vi "Part 2.vi"(11 "Input":string) -> (3 "Output":i64)   [LabVIEW 2021]
uses:
  <userlib>/_OpenG.lib/string/string.llb/Convert EOLs (String)__ogtk.vi
  0a5bc26e-a1a3-4762-95bb-f84fbea421ee.vi
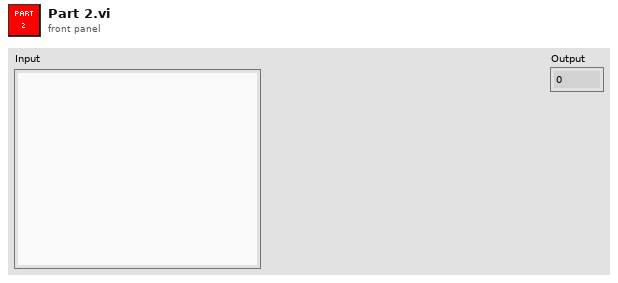
[diagram p1: front panel]
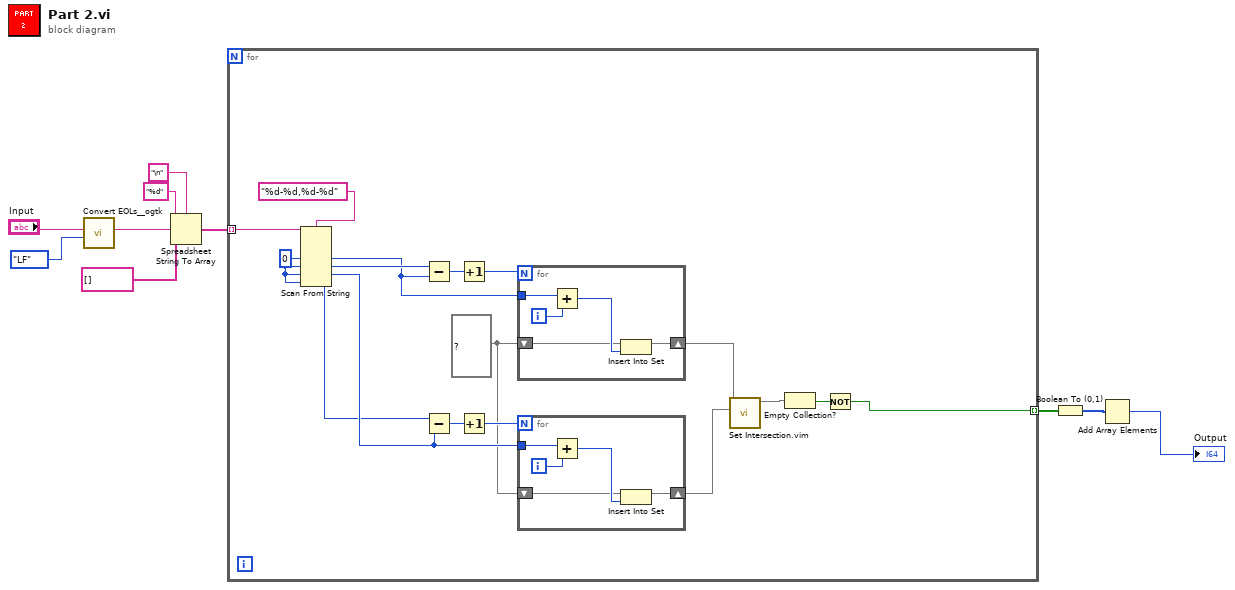
[diagram p0: block diagram]
diagram:
  n1 = call-poly <userlib>:"Convert EOLs__ogtk.vi"("Convert to:"=enum16{"CR", "LF", "CRLF"}."LF", "String in"="Input") -> ("String out"=w7:string)  [unwired: 9 in]
  n2 = Spreadsheet String To Array(delimiter (Tab)="\n", format string="%d", spreadsheet string=w7, array type (2D Dbl)=string[] []) -> (array=w5:string[])
  n3 = for {
    tunnel: w5 -> [w27] mode=indexing
    tunnel: [w11] -> w4 mode=indexing
    w16 = set{i64} {} ("set out")
    w25 = i64 0 ("default value 1")
    n4 = Scan From String(format string="%d-%d,%d-%d", input string=w27, default 1=w25, default 2=w25, default 3=w25, default 4=w25) -> (output 1=w21:i64, output 2=w24:i64, output 3=w19:i64, output 4=w18:i64)  [unwired: 2 in, 3 out]
    n5 = Subtract(x=w24, y=w21) -> (x-y=w23:i64)
    n6 = Subtract(x=w18, y=w19) -> (x-y=w20:i64)
    n7 = Increment(x=w23) -> (x+1=w22:i64)
    n8 = Increment(x=w20) -> (x+1=w17:i64)
    n9 = for {
      N: w22 -> [_]
      tunnel: w21 -> [w37]
      shift-right: [w33] -> w15
      shift-left: w16 -> [w34]
      i -> [w36]
      n10 = Add(x=w37, y=w36) -> (x+y=w35:i64)
      n11 = Insert Into Set(10:w35, 11:w34) -> (3:w33:set{i64})  [unwired: 1 out]
    }
    n12 = for {
      N: w17 -> [_]
      tunnel: w19 -> [w32]
      shift-right: [w28] -> w14
      shift-left: w16 -> [w29]
      i -> [w31]
      n13 = Add(x=w32, y=w31) -> (x+y=w30:i64)
      n14 = Insert Into Set(10:w30, 11:w29) -> (3:w28:set{i64})  [unwired: 1 out]
    }
    n15 = call "Set Intersection.vim"("set 2"=w14, "set 1"=w15) -> ("intersection"=w13:set{i64})  [unwired: 9 in]
    n16 = Empty Collection?(1:w13) -> (0:w12:bool)
    n17 = Not(x=w12) -> (.not. x?=w11:bool)
  }
  n18 = Boolean To (0,1)(Boolean=w4) -> (0, 1=w3:i16[])
  n19 = Add Array Elements(numeric array=w3) -> (sum=→"Output":i16)
